vi "Write to DigiSrc file.vi"(8 "error in (no error)":errorcluster, 10 "Pattern  Contents":string, 11 "Pattern Name":string) -> (0 "error out":errorcluster, 3 "DigiSrc File":path)   [LabVIEW 2018]
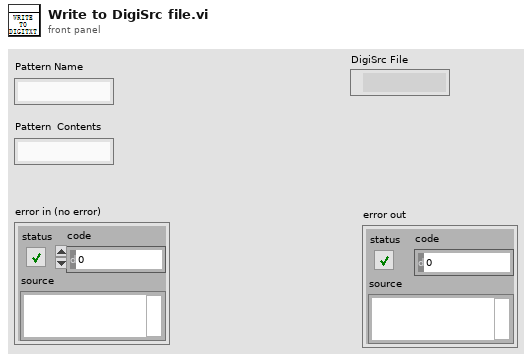
[diagram p1: front panel]
types:
  T1 = enum16{"open", "replace", "create", "open or create", "replace or create", "replace or create with confirmation"}
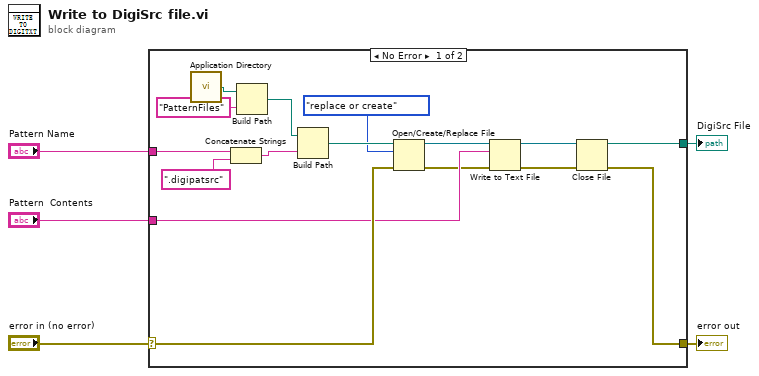
[diagram p0: block diagram]
diagram:
  n1 = case shown="No Error" "error in (no error)" {
    selector: "error in (no error)" -> [w17 w22]
    tunnel: "Pattern Name" -> [w8 _]
    tunnel: "Pattern  Contents" -> [w14 _]
    tunnel: [w10 w22] -> w2
    tunnel: [w9 _] -> w1
    frame No Error {
      n2 = call <vilib>:"Application Directory.vi"() -> ("Application Directory"=w21:path)
      n3 = Concatenate Strings(w8, ".digipatsrc" ("string")) -> (w7:string)
      n4 = Build Path(base path=w21, name or relative path="PatternFiles") -> (appended path=w19:path)
      n5 = Build Path(base path=w19, name or relative path=w7) -> (appended path=w18:path)
      n6 = Open/Create/Replace File(file path (use dialog)=w18, error in=w17, operation (0:open)=T1."replace or create") -> (refnum out=w15:refnum<file>, error out=w13:errorcluster)  [unwired: 3 in, 1 out]
      n7 = Write to Text File(file (use dialog)=w15, text=w14, error in=w13) -> (refnum out=w12:refnum<file>, error out=w11:errorcluster)  [unwired: 1 in, 1 out]
      n8 = Close File(refnum=w12, error in=w11) -> (path=w9:path, error out=w10:errorcluster)
    }
    frame Error {
    }
  }
  "error out" <- w2
  "DigiSrc File" <- w1
